vi "test Anchor Array to Cluster Array.vi"(8 "error in (no error)":errorcluster, 11 "TestCase in":refnum<class "AnchorTests.lvclass">) -> (0 "error out":errorcluster, 3 "TestCase out":refnum<class "AnchorTests.lvclass">)   [LabVIEW 2014, in "AnchorTests.lvclass"]
uses:
  AnchorTests.lvclass
  SPLAT/Anchor/Anchor.lvclass
  <vilib>/addons/_JKI Toolkits/VI Tester/TestCase.llb/TestCase.lvclass
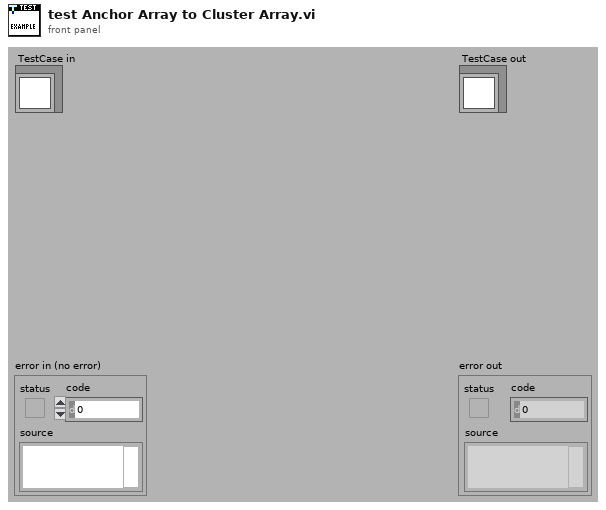
[diagram p1: front panel]
types:
  T1 = cluster{"AnchorID":dbl, "AnchorX":dbl, "AnchorY":dbl}[]
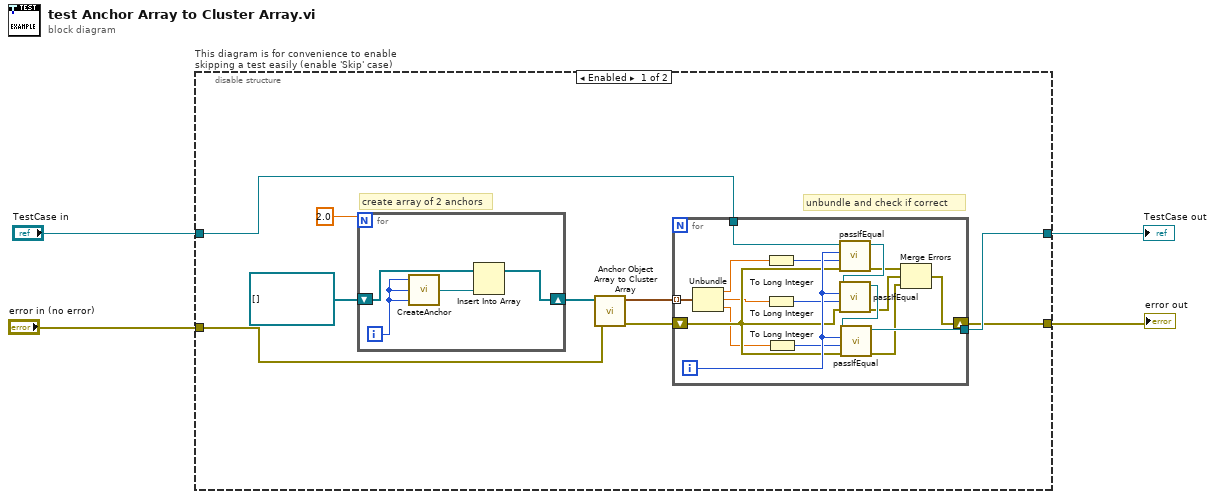
[diagram p0: block diagram]
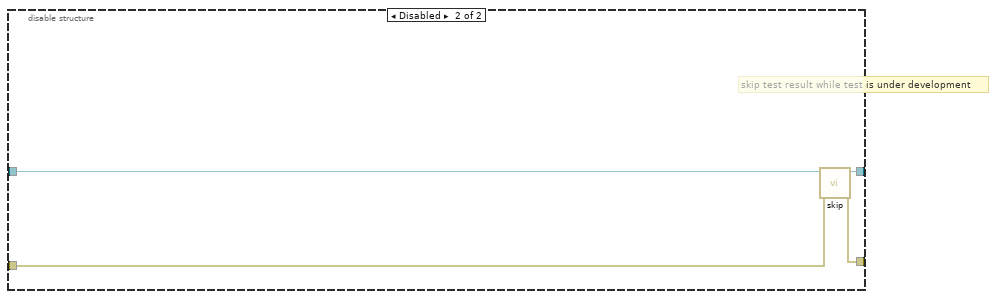
[diagram p2: hidden frame]
diagram:
  n1 = disable-structure "This diagram is for convenience to enable skipping a test easily (enable 'Skip' case)" shown="Enabled" {
    disable-tunnel: "TestCase in" -> [w8 w38]
    disable-tunnel: [w7 w36] -> w1
    disable-tunnel: [w5 w37] -> w3
    disable-tunnel: "error in (no error)" -> [w10 w35]
    frame Enabled {
      # "unbundle and check if correct"
      # "create array of 2 anchors"
      n2 = for {
        N: 2.0 -> [_]
        shift-right: [w31] -> w11
        shift-left: refnum<class "Anchor.lvclass">[] [] -> [w34]
        i -> [w33]
        n3 = call "CreateAnchor.vi"("Anchor Y"=w33, "Anchor X"=w33, "Anchor ID"=w33) -> ("Anchor Out"=w32:refnum<class "Anchor.lvclass">)
        n4 = Insert Into Array(array=w34, new element=w32) -> (w31:refnum<class "Anchor.lvclass">[])  [unwired: 1 in]
      }
      n5 = call "Anchor Object Array to Cluster Array.vi"("error in (no error)"=w10, "AnchorArray In"=w11) -> ("error out"=w6:errorcluster, "AnchorArray Out"=w9:T1)  [unwired: 8 in]
      n6 = for {
        tunnel: w9 -> [w30] mode=indexing
        tunnel: w8 -> [w28]
        tunnel: [w25] -> w7
        shift-right: [w20] -> w5
        shift-left: w6 -> [w21]
        i -> [w29]
        n7 = Unbundle(w30) -> ("AnchorID"=w19:dbl, "AnchorX"=w17:dbl, "AnchorY"=w15:dbl)
        n8 = To Long Integer(number=w19) -> (32bit integer=w18:i32)
        n9 = To Long Integer(number=w17) -> (32bit integer=w16:i32)
        n10 = To Long Integer(number=w15) -> (32bit integer=w14:i32)
        n11 = call-dynamic "passIfEqual.vi"("error in (no error)"=w21, "y"=w18, "x"=w29, "TestCase in"=w28) -> ("error out"=w24:errorcluster, "TestCase out"=w27:refnum<class "AnchorTests.lvclass">)  [unwired: 6 in]
        n12 = call-dynamic "passIfEqual.vi"("error in (no error)"=w21, "y"=w16, "x"=w29, "TestCase in"=w27) -> ("error out"=w23:errorcluster, "TestCase out"=w26:refnum<class "AnchorTests.lvclass">)  [unwired: 6 in]
        n13 = call-dynamic "passIfEqual.vi"("error in (no error)"=w21, "y"=w14, "x"=w29, "TestCase in"=w26) -> ("error out"=w22:errorcluster, "TestCase out"=w25:refnum<class "AnchorTests.lvclass">)  [unwired: 6 in]
        n14 = Merge Errors(w24, w23, w22) -> (w20:errorcluster)
      }
    }
    frame Disabled {
      # "skip test result while test is under development"
      n15 = call <vilib>:"skip.vi"("error in (no error)"=w35, "TestCase in"=w38) -> ("error out"=w37:errorcluster, "TestCase out"=w36:refnum<class "AnchorTests.lvclass">)  [unwired: 8 in]
    }
  }
  "error out" <- w3
  "TestCase out" <- w1
